vi "G# - InterfaceDemo4.vi"() -> ()   [LabVIEW 2020]
doc: "G# Interface Implementation\nThis examples demonstrates how to use the G#Interface. The interface concept is an alternative design principle to multiple inheritance (just as in C# and Java). Classes that are not related can implement the same interface and the reference of the interface could be treated just as they are from the same class.\n\nBy using the G# Debugger found in Tools->G# Debugger a text log can be followed showing how the objects were created and destroyed."
uses:
  IMyInterface3_interface/IMyInterface3.lvclass
  MyClass6_class/MyClass6.lvclass
  C:/Program Files (x86)/National Instruments/LabVIEW 2020/examples/AddQ/G#/Interface/IMyInterface3_interface/IMyInterface3.lvclass
  MyClass5_class/MyClass5.lvclass
  <vilib>/addons/_AddQ/G#Object/G#Object.lvclass
panel:
  out "# of objects killed":i32
  out "OK":bool
  in  "error in (no error)":errorcluster
  out "MyClass6 is instance of IMyInterface4":bool
  out "MyClass5 is instance of IMyInterface3":bool
  out "error out":errorcluster
  out "Class Name":string[](array[string])
  # "G# Interface Implementation native Interface in LV2020\nThis examples demonstrates how to use the native interface in LV2020 with G#. Classes that are not related can implement the same interface\nand the reference of the interface could be treated just as they are from the same class.\n\nBy using the G# Debugger found in Tools->G# Debugger a text log can be followed showing how the objects were created and destroyed."
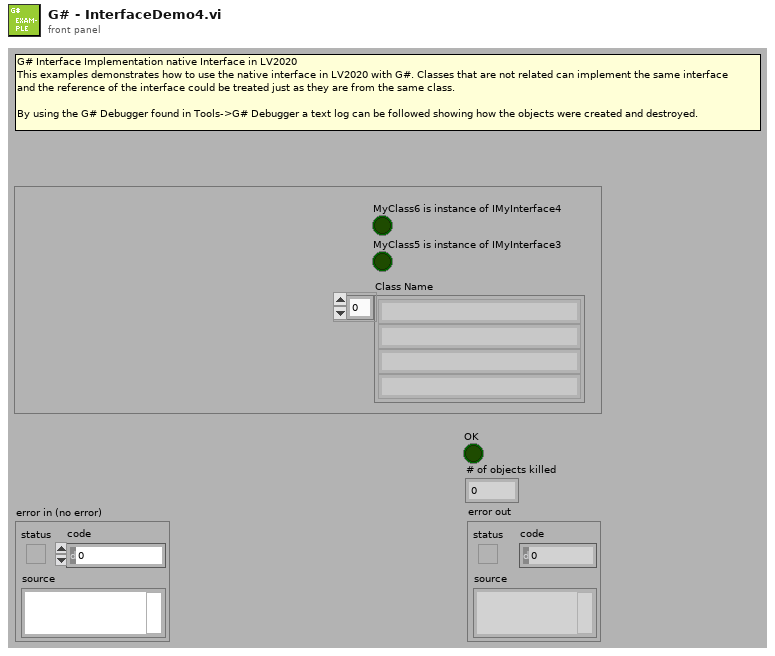
[diagram p1: front panel]
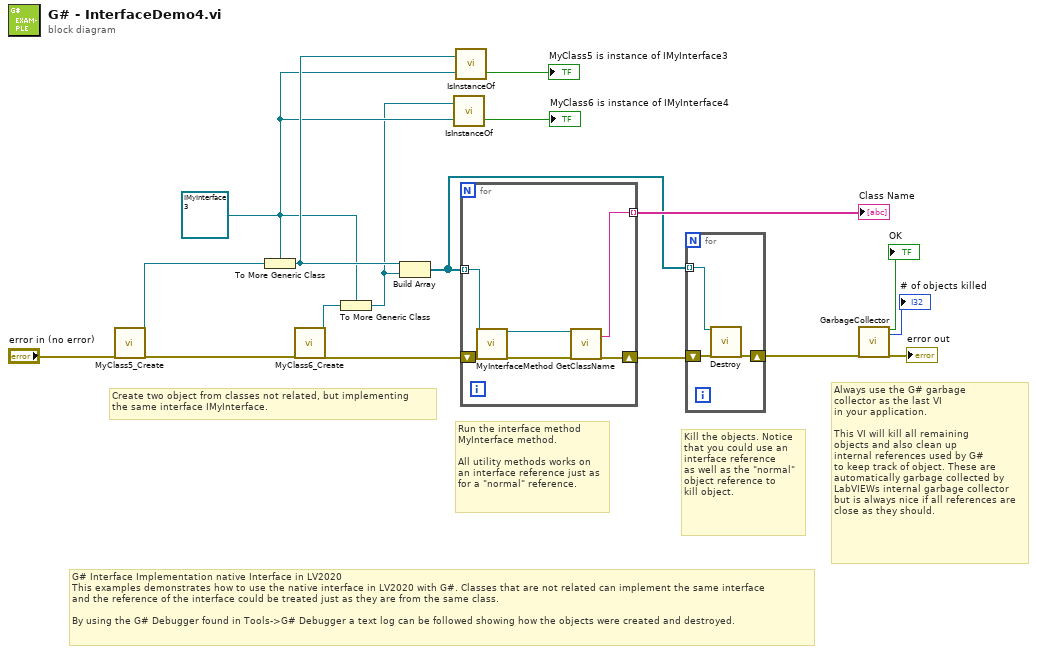
[diagram p0: block diagram]
diagram:
  w3 = refnum<class "IMyInterface3.lvclass"> refnum ("IMyInterface3")
  # "G# Interface Implementation native Interface in LV2020\nThis examples demonstrates how to use the native interface in LV2020 with G#. Classes that are not related can implement the same interface\nand the reference of the interface could be treated just as they are from the same class.\n\nBy using the G# Debugger found in Tools->G# Debugger a text log can be followed showing how the objects were created and destroyed."
  # "Always use the G# garbage\ncollector as the last VI\nin your application.\n\nThis VI will kill all remaining\nobjects and also clean up\ninternal references used by G#\nto keep track of object. These are\nautomatically garbage collected by\nLabVIEWs internal garbage collector\nbut is always nice if all references are\nclose as they should."
  # "Kill the objects. Notice\nthat you could use an\ninterface reference\nas well as the \"normal\"\nobject reference to\nkill object."
  # "Run the interface method\nMyInterface method.\n\nAll utility methods works on\nan interface reference just as\nfor a \"normal\" reference."
  # "Create two object from classes not related, but implementing\nthe same interface IMyInterface."
  n1 = call "MyClass5_Create.vi"("error in (no error)"="error in (no error)") -> ("reference out"=w8:refnum<class "MyClass5.lvclass">, "error out"=w10:errorcluster)  [unwired: 17 in]
  n2 = To More Generic Class(target class=w3, reference=w8) -> (generic class reference=w5:refnum<class "IMyInterface3.lvclass">)
  n3 = call "MyClass6_Create.vi"("error in (no error)"=w10) -> ("reference out"=w7:refnum<class "MyClass6.lvclass">, "error out"=w9:errorcluster)  [unwired: 17 in]
  n4 = To More Generic Class(target class=w3, reference=w7) -> (generic class reference=w2:refnum<class "IMyInterface3.lvclass">)
  n5 = Build Array(w5, w2) -> (w6:refnum<class "IMyInterface3.lvclass">[])
  n6 = call-dynamic "IsInstanceOf.vi"("is object instance of"=w3, "reference in"=w2) -> ("is instance of"=→"MyClass6 is instance of IMyInterface4":bool)  [unwired: 1 out]
  n7 = call-dynamic "IsInstanceOf.vi"("is object instance of"=w3, "reference in"=w5) -> ("is instance of"=→"MyClass5 is instance of IMyInterface3":bool)  [unwired: 1 out]
  n8 = for {
    shift-right: [w21] -> w16
    shift-left: w9 -> [w23]
    tunnel: w6 -> [w22] mode=indexing
    tunnel: [w20] -> w15 mode=indexing
    n9 = call-dynamic "MyInterfaceMethod.vi"("reference in"=w22, "error in (no error)"=w23) -> ("reference out"=w19:refnum<class "IMyInterface3.lvclass">, "error out"=w18:errorcluster)  [unwired: 16 in]
    n10 = call-dynamic "GetClassName.vi"("reference in"=w19, "error in (no error)"=w18) -> ("class name"=w20:string, "error out"=w21:errorcluster)  [unwired: 13 in, 3 out]
  }
  "Class Name" <- w15
  n11 = for {
    shift-right: [w25] -> w14
    shift-left: w16 -> [w26]
    tunnel: w6 -> [w24] mode=indexing
    n12 = call-dynamic "Destroy.vi"("reference in"=w24, "error in (no error)"=w26) -> ("error out"=w25:errorcluster)  [unwired: 16 in, 1 out]
  }
  n13 = call <vilib>:"GarbageCollector.vi"("error in (no error)"=w14) -> ("OK"=→"OK":bool, "# of objects killed"=→"# of objects killed":i32, "error out"=→"error out":errorcluster)  [unwired: 16 in]
